vi "Bring Window Forward (WinAPI).vi"(8 "error in (no error)":errorcluster, 11 "VI reference in":refnum<vi>) -> (0 "error out":errorcluster, 1 "Handle":u64, 3 "VI reference out":refnum<vi>)   [LabVIEW 2017]
doc: "Brings the window of VI reference in to the foreground and gives it the keyboard focus, using the Win32 SetForegroundWindow API. The window handle is returned."
uses:
  USER32.DLL
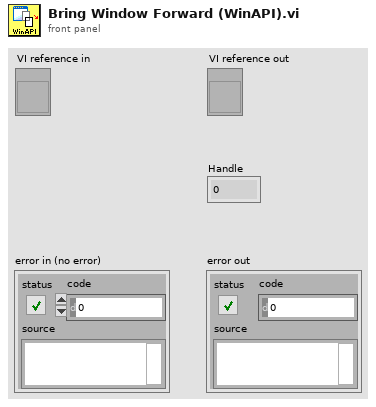
[diagram p1: front panel]
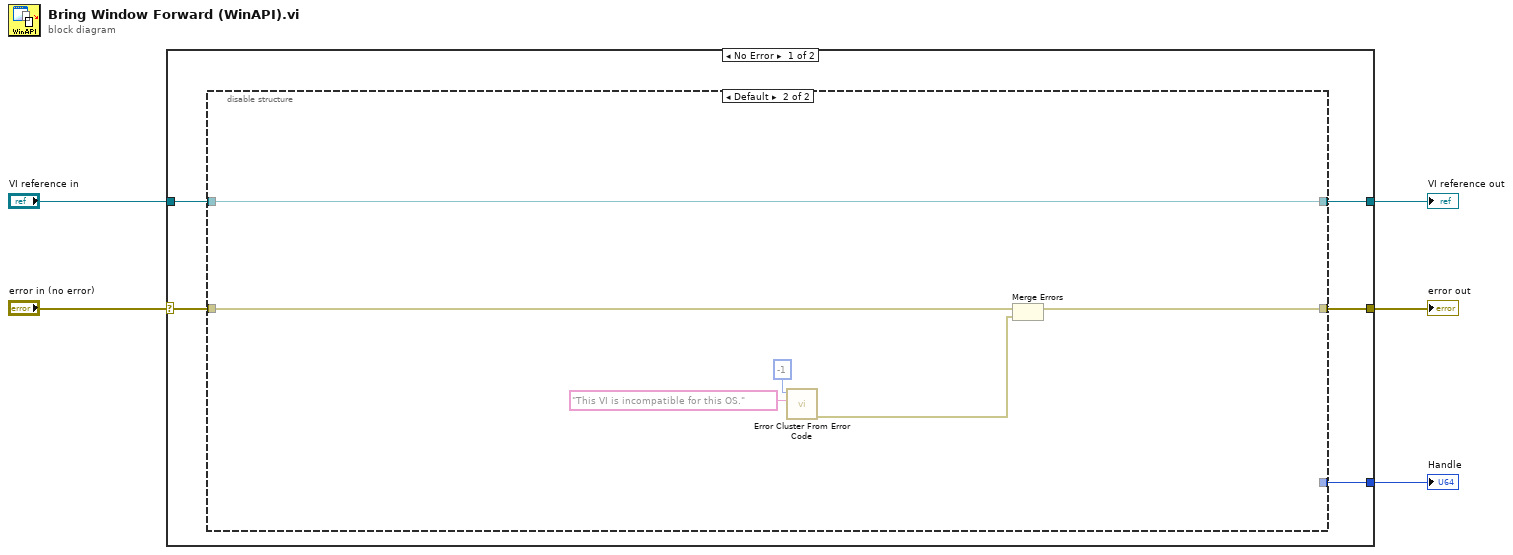
[diagram p0: block diagram]
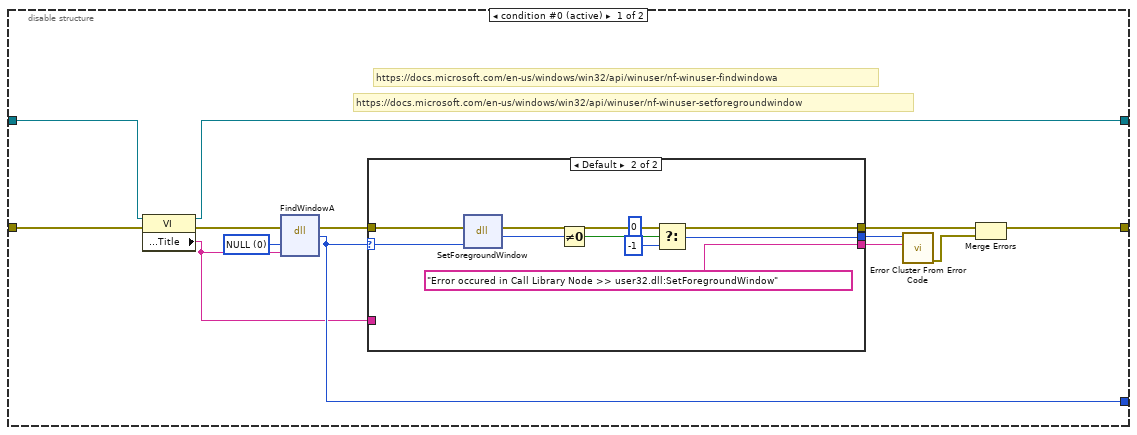
[diagram p2: hidden frame]
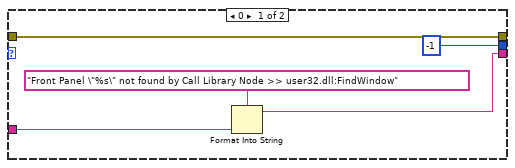
[diagram p3: hidden frame]
diagram:
  n1 = case shown="No Error" "error in (no error)" {
    selector: "error in (no error)" -> [w8 w45]
    tunnel: [w7 w45] -> w5
    tunnel: [w6 _] -> w4
    tunnel: [w10 w44] -> w3
    tunnel: "VI reference in" -> [w9 w44]
    frame No Error {
      n2 = disable-structure shown="Default" {
        disable-tunnel: [w19 w43] -> w10
        disable-tunnel: w9 -> [w18 w43]
        disable-tunnel: w8 -> [w17 w40]
        disable-tunnel: [w16 w39] -> w7
        disable-tunnel: [w15 _] -> w6
        frame condition #0 (active) {
          w21 = 0 items=["NULL"]
          # "https://docs.microsoft.com/en-us/windows/win32/api/winuser/nf-winuser-findwindowa"
          # "https://docs.microsoft.com/en-us/windows/win32/api/winuser/nf-winuser-setforegroundwindow"
          n3 = property class="VI"(reference=w18, error in=w17) -> (reference out=w19:refnum<vi>, error out=w20:errorcluster, "Front Panel.Title"=w11:string)
          n4 = dll-call lib="user32.dll" fn="FindWindowA"(error in=w20, "lpszClassName"=w21, "lpszWindowName"=w11) -> (error out=w22:errorcluster, "hWnd"=w15:u64)  [unwired: 3 in, 2 out]
          n5 = case shown="Default" w15 {
            selector: w15 -> [_ w34]
            tunnel: [w28 w37] -> w23
            tunnel: w22 -> [w28 w36]
            tunnel: [-1 ("return type") w32] -> w13
            tunnel: [w25 "Error occured in Call Library Node >> user32.dll:SetForegroundWindow" ("error message (\"\")")] -> w12
            tunnel: w11 -> [w24 _]
            frame 0 {
              n6 = Format Into String(format string="Front Panel \"%s\" not found by Call Library Node >> user32.dll:FindWindow" ("error message (\"\")"), w24) -> (resulting string=w25:string)  [unwired: 2 in, 1 out]
            }
            frame Default {
              n7 = dll-call lib="USER32.DLL" fn="SetForegroundWindow"(error in=w36, "Handle"=w34) -> (error out=w37:errorcluster, "return type"=w31:i32)  [unwired: 3 in, 1 out]
              n8 = Not Equal To 0?(x=w31) -> (x != 0?=w33:bool)
              n9 = Select(t=0, s=w33, f=-1) -> (s? t:f=w32:i32)
            }
          }
          n10 = call <vilib>:"Error Cluster From Error Code.vi"("error message (\"\")"=w12, "error code (0)"=w13) -> ("error out"=w14:errorcluster)  [unwired: 7 in]
          n11 = Merge Errors(w23, w14) -> (w16:errorcluster)
        }
        frame condition #1 {
          n12 = call <vilib>:"Error Cluster From Error Code.vi"("error message (\"\")"="This VI is incompatible for this OS." ("error message (\"\")"), "error code (0)"=-1) -> ("error out"=w38:errorcluster)  [unwired: 7 in]
          n13 = Merge Errors(w40, w38) -> (w39:errorcluster)
        }
      }
    }
    frame Error {
    }
  }
  "Handle" <- w4
  "error out" <- w5
  "VI reference out" <- w3
